vi "Retriger_Sequence.vi"(7 "Filename (.ini)":string="Config_Ver_1\\pulse_sequence.ini", 8 "error in":errorcluster, 11 "VISA arduino in":refnum<visa-resource-name>) -> (0 "error out":errorcluster, 1 "register 2 (8-13)":T2, 2 "register 1 (2-7)":T3, 3 "VISA arduino out":refnum<visa-resource-name>, 5 "Pulse sequence":T1[](array[typedef]) {"channel" min=2 max=13 step=1})   [LabVIEW 2021]
uses:
  Drivers/Arduino_Pulse_Generator/Configurate/Register_1.ctl
  Drivers/Arduino_Pulse_Generator/Configurate/Register_2.ctl
  Drivers/Arduino_Pulse_Generator/Configurate/Channel_Pulse_Stream.ctl
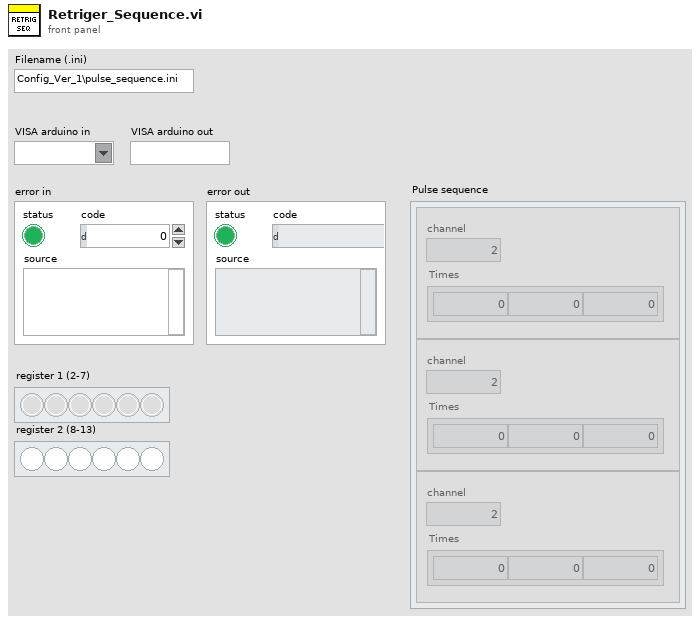
[diagram p1: front panel]
types:
  T1 = typedef "Channel_Pulse_Stream.ctl" = cluster{"Times":dbl[], "channel":u8}
  T2 = typedef "Register_2.ctl" = bool[]
  T3 = typedef "Register_1.ctl" = bool[]
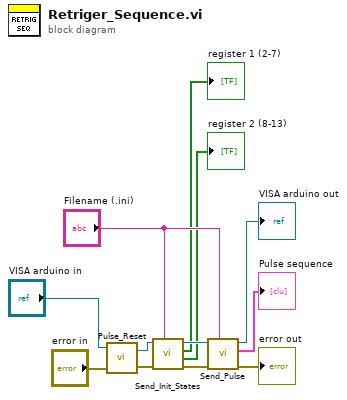
[diagram p0: block diagram]
diagram:
  n1 = call "Pulse_Reset.vi"("error in"="error in", "VISA arduino in"="VISA arduino in") -> ("error out"=w11:errorcluster, "VISA arduino out"=w12:refnum<visa-resource-name>)  [unwired: 1 in]
  n2 = call "Send_Init_States.vi"("Filename (.ini)"="Filename (.ini)", "error in"=w11, "VISA arduino in"=w12) -> ("error out"=w9:errorcluster, "register 2 (8-13)"=→"register 2 (8-13)":T2, "register 1 (2-7)"=→"register 1 (2-7)":T3, "VISA arduino out"=w10:refnum<visa-resource-name>)  [unwired: 5 in]
  n3 = call "Send_Pulse.vi"("Filename (.ini)"="Filename (.ini)", "error in"=w9, "VISA arduino in"=w10) -> ("error out"=→"error out":errorcluster, "Pulse sequence"=→"Pulse sequence":T1[], "VISA arduino out"=→"VISA arduino out":refnum<visa-resource-name>)  [unwired: 6 in]
